vi "Close Instrument.vi"(7 "Go Local (\"@LOC\")":bool, 8 "error in (no error)":errorcluster, 11 "NI USB-6501 in":refnum<class "NI USB-6501.lvclass">) -> (0 "error out":errorcluster, 3 "NI USB-6501 out":refnum<class "NI USB-6501.lvclass">)   [LabVIEW 2020, in "NI USB-6501.lvclass"]
uses:
  NI USB-6501.lvclass
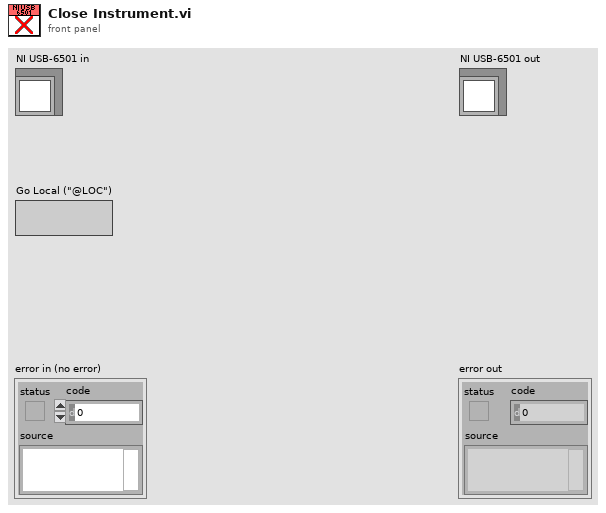
[diagram p1: front panel]
types:
  T1 = typedef "NI USB-6501.lvclass/Channel.ctl" = cluster{"Channel":tag, "Task":refnum<k21>, "Function":string, "Low":string, "High":string, "Direction":enum16{"Input", "Output"}}
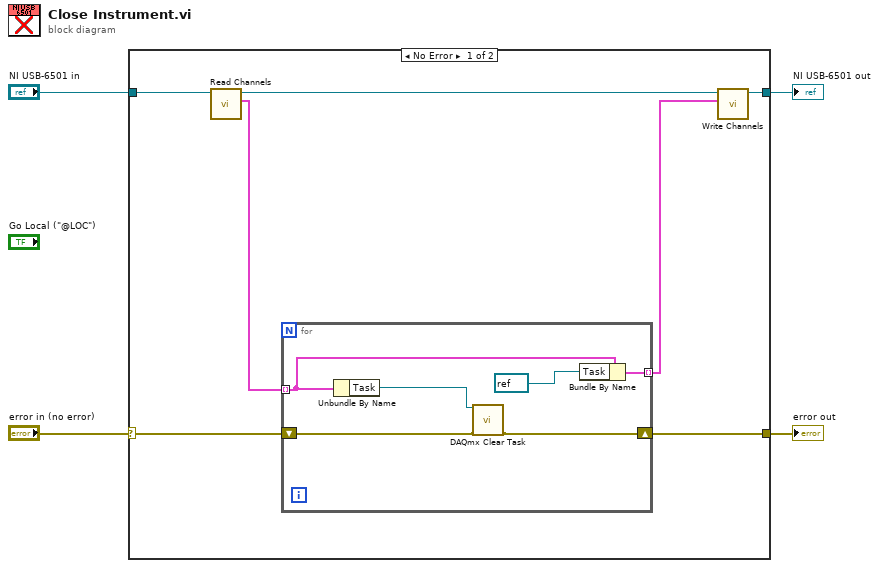
[diagram p0: block diagram]
diagram:
  n1 = case shown="No Error" "error in (no error)" {
    selector: "error in (no error)" -> [w7 w19]
    tunnel: [w8 w19] -> w4
    tunnel: "NI USB-6501 in" -> [w11 w18]
    tunnel: [w5 w18] -> w3
    frame No Error {
      n2 = call-dynamic "Read Channels.vi"("NI USB-6501 in"=w11) -> ("Channels"=w9:T1[], "NI USB-6501 out"=w10:refnum<class "NI USB-6501.lvclass">)  [unwired: 9 in]
      n3 = for {
        tunnel: w9 -> [w17] mode=indexing
        shift-right: [w14] -> w8
        shift-left: w7 -> [w15]
        tunnel: [w16] -> w6 mode=indexing
        n4 = Unbundle By Name(w17) -> ("Task"=w13:refnum<k21>)
        n5 = call <vilib>:"DAQmx Clear Task.vi"("task in"=w13, "error in"=w15) -> ("error out"=w14:errorcluster)  [unwired: 13 in]
        n6 = Bundle By Name(cluster=w17, "Task"=refnum<k21> refnum) -> (w16:T1)
      }
      n7 = call-dynamic "Write Channels.vi"("Channels"=w6, "NI USB-6501 in"=w10) -> ("NI USB-6501 out"=w5:refnum<class "NI USB-6501.lvclass">)  [unwired: 9 in]
    }
    frame Error {
    }
  }
  "error out" <- w4
  "NI USB-6501 out" <- w3
